vi "Main.vi"(8 "error in (no error)":errorcluster, 10 "Status  Monitor":string, 11 "Result Display in":refnum<class "Result Display.lvclass">) -> (0 "error out":errorcluster, 3 "Result Display out":refnum<class "Result Display.lvclass">)   [LabVIEW 2018, in "Result Display.lvclass"]
uses:
  Result Display.lvclass
  UI Interface.vi
  Process Bar/Process Bar.lvclass
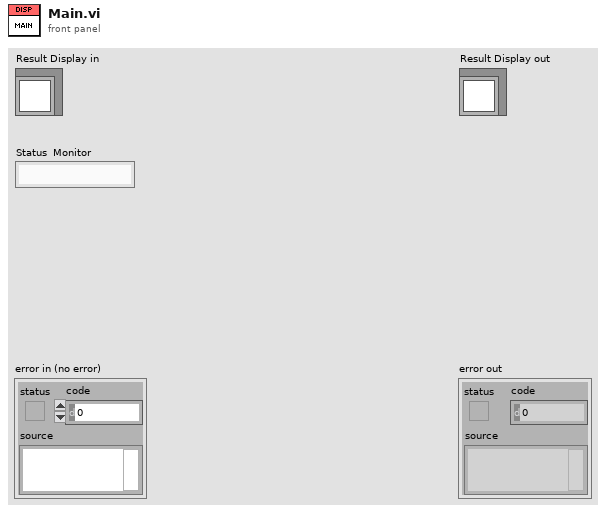
[diagram p1: front panel]
types:
  T1 = enum32{"Invalid", "Standard", "Closed", "Hidden", "Minimized", "Maximized"}
  T2 = typedef "Process Bar.lvclass/Session Handle.ctl" = refnum<data-value>
  T3 = typedef "Result Data Mgr.lvclass/GRR Result.ctl" = cluster{"Test Name":string, "Parts #":u8, "Appraiser #":u8, "Trial #":u8, "Percent AV":dbl, "Percent EV":dbl, "Percent GRR":dbl}
  T4 = typedef "TestDataMgr.lvclass/Test Data All.ctl" = cluster{"Test Name":string, "Test Limits":T5, "Raw Data Per Tester":T6[]}
  T5 = typedef "TestDataMgr.lvclass/Test Limits.ctl" = cluster{"High":dbl, "Low":dbl}
  T6 = typedef "TestDataMgr.lvclass/Test Raw Data.ctl" = cluster{"Data":dbl[][], "Tester#":u8}
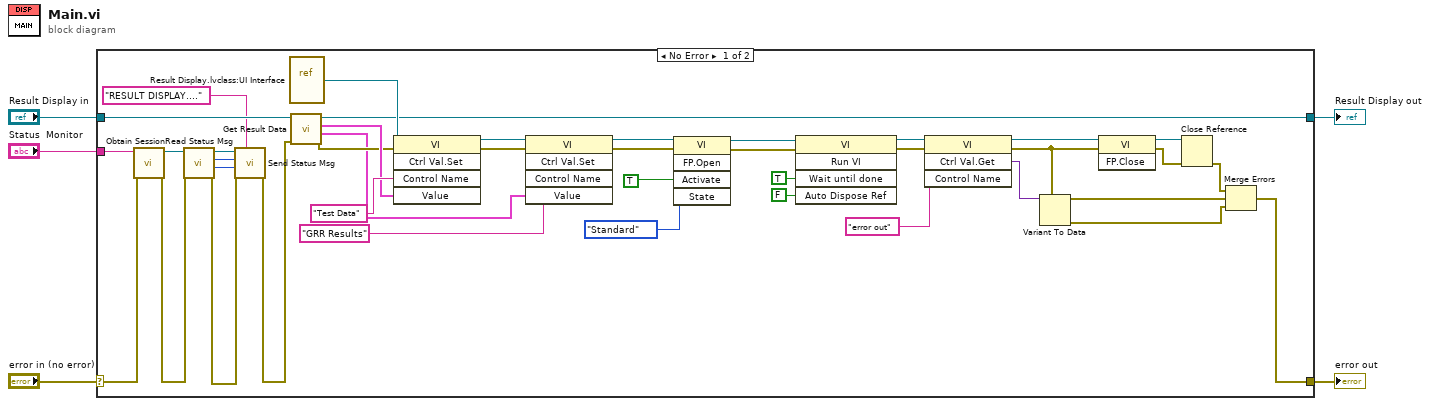
[diagram p0: block diagram]
diagram:
  n1 = case shown="No Error" "error in (no error)" {
    selector: "error in (no error)" -> [w15 w47]
    tunnel: [w22 w47] -> w4
    tunnel: [w21 w46] -> w2
    tunnel: "Result Display in" -> [w45 w46]
    tunnel: "Status  Monitor" -> [w14 _]
    frame No Error {
      n2 = call "Obtain Session.vi"("error in (no error)"=w15, "Session  Name ()"=w14) -> ("error out"=w7:errorcluster, "Session Handle"=w11:T2)  [unwired: 8 in]
      n3 = call "Read Status Msg.vi"("error in (no error)"=w7, "Session Handle in"=w11) -> ("error out"=w6:errorcluster, "Process Max"=w8:u16, "Process Bar"=w9:u8, "Session Handle out"=w10:T2)  [unwired: 5 in, 1 out]
      n4 = call "Send Status Msg.vi"("Status Msg"="RESULT DISPLAY....", "error in (no error)"=w6, "Process Max"=w8, "Process Bar"=w9, "Session Handle in"=w10) -> ("error out"=w13:errorcluster)  [unwired: 5 in, 1 out]
      n5 = vi-ref "Result Display.lvclass:UI Interface.vi"() -> (w42:refnum<vi>)
      n6 = call "Get Result Data.vi"("error in (no error)"=w13, "Result Display in"=w45) -> ("error out"=w39:errorcluster, "GRR Results"=w35:T3[], "Test Data"=w40:T4[], "Result Display out"=w21:refnum<class "Result Display.lvclass">)  [unwired: 6 in]
      n7 = invoke class="VI" method="Ctrl Val.Set"(reference=w42, error in=w39, "Control Name"="Test Data", "Value"=w40) -> (reference out=w38:refnum<vi>, error out=w37:errorcluster)  [unwired: 1 in, 3 out]
      n8 = invoke class="VI" method="Ctrl Val.Set"(reference=w38, error in=w37, "Control Name"="GRR Results", "Value"=w35) -> (reference out=w34:refnum<vi>, error out=w33:errorcluster)  [unwired: 1 in, 3 out]
      n9 = invoke class="VI" method="FP.Open"(reference=w34, error in=w33, "Activate"=TRUE ("Activate?"), "State"=T1."Standard") -> (reference out=w32:refnum<vi>, error out=w31:errorcluster)  [unwired: 1 in, 3 out]
      n10 = invoke class="VI" method="Run VI"(reference=w32, error in=w31, "Wait until done"=TRUE ("Wait Until Done"), "Auto Dispose Ref"=FALSE ("Auto Dispose Reference")) -> (reference out=w28:refnum<vi>, error out=w27:errorcluster)  [unwired: 1 in, 3 out]
      n11 = invoke class="VI" method="Ctrl Val.Get"(reference=w28, error in=w27, "Control Name"="error out") -> (reference out=w20:refnum<vi>, error out=w19:errorcluster, "Get Control Value Variant"=w25:variant)  [unwired: 1 in, 1 out]
      n12 = Variant To Data(type=w19, Variant=w25) -> (data=w24:errorcluster, error out=w23:errorcluster)  [unwired: 1 in]
      n13 = invoke class="VI" method="FP.Close"(reference=w20, error in=w19) -> (reference out=w18:refnum<vi>, error out=w17:errorcluster)  [unwired: 1 in, 1 out]
      n14 = Close Reference(reference=w18, error in (no error)=w17) -> (error out=w16:errorcluster)
      n15 = Merge Errors(w16, w24, w23) -> (w22:errorcluster)
    }
    frame Error {
    }
  }
  "error out" <- w4
  "Result Display out" <- w2
